vi "ConvertGP354InputBytes.vi"(11 "GP354 Bytes":u8[](array[numeric])) -> (3 "Pressure":dbl)   [LabVIEW 2011]
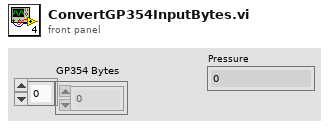
[diagram p1: front panel]
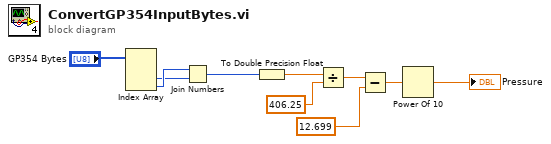
[diagram p0: block diagram]
diagram:
  n1 = Index Array(array="GP354 Bytes") -> (element #2=w2:u8, element #3=w3:u8)  [unwired: 3 in, 1 out]
  n2 = Join Numbers(hi=w3, lo=w2) -> ((hi.lo)=w4:u16)
  n3 = To Double Precision Float(number=w4) -> (double precision float=w5:dbl)
  n4 = Divide(x=w5, y=406.25) -> (x/y=w9:dbl)
  n5 = Subtract(x=w9, y=12.699) -> (x-y=w7:dbl)
  n6 = Power Of 10(x=w7) -> (10^x=→"Pressure":dbl)
